vi "Distance.vi"(8 "error in (no error)":errorcluster, 9 "P1":dbl[](array[numeric]), 10 "P2":dbl[](array[numeric]), 11 "Utilities in":refnum<class "Utilities.lvclass">) -> (0 "error out":errorcluster, 2 "Distance":dbl, 3 "Utilities out":refnum<class "Utilities.lvclass">)   [LabVIEW 2023, in "Utilities.lvclass"]
uses:
  Utilities.lvclass
  Utilities.lvclass/Utilities.ctl
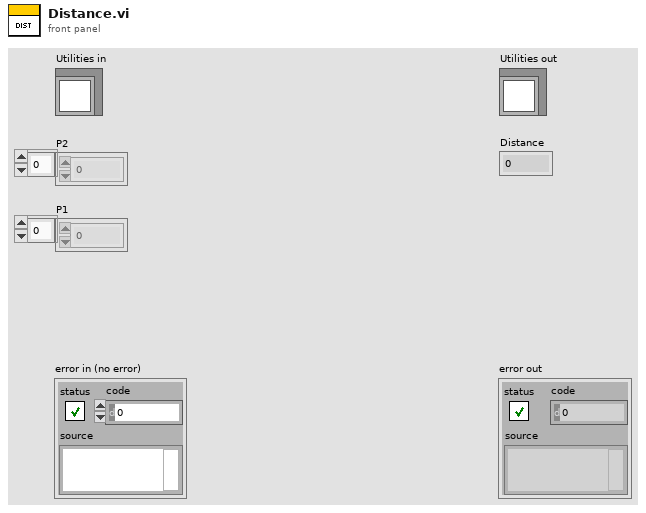
[diagram p1: front panel]
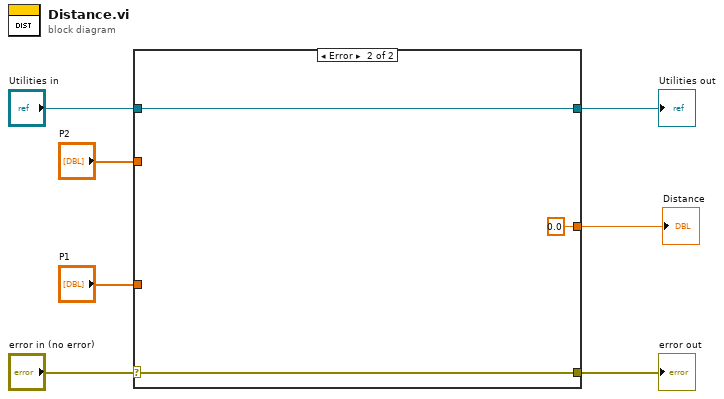
[diagram p0: block diagram]
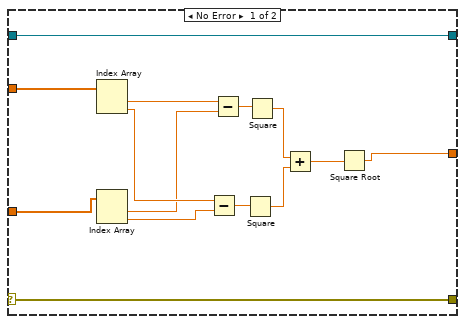
[diagram p2: hidden frame]
diagram:
  n1 = case shown="Error" "error in (no error)" {
    selector: "error in (no error)" -> [w20 w24]
    tunnel: [w20 w24] -> w6
    tunnel: [w21 w23] -> w4
    tunnel: "Utilities in" -> [w21 w23]
    tunnel: "P2" -> [w12 _]
    tunnel: "P1" -> [w11 _]
    tunnel: [w8 0.0] -> w1
    frame No Error {
      n2 = Index Array(array=w12) -> (element #1=w19:dbl, element #2=w18:dbl)  [unwired: 2 in]
      n3 = Index Array(array=w11) -> (element #1=w10:dbl, element #2=w9:dbl)  [unwired: 2 in]
      n4 = Subtract(x=w18, y=w9) -> (x-y=w16:dbl)
      n5 = Subtract(x=w19, y=w10) -> (x-y=w17:dbl)
      n6 = Square(x=w16) -> (x^2=w14:dbl)
      n7 = Square(x=w17) -> (x^2=w15:dbl)
      n8 = Add(x=w15, y=w14) -> (x+y=w13:dbl)
      n9 = Square Root(x=w13) -> (sqrt(x)=w8:dbl)
    }
    frame Error {
    }
  }
  "error out" <- w6
  "Utilities out" <- w4
  "Distance" <- w1
